vi "PLC Driver.vi"(0 "Data Cluster":T2={"Baud Rate"=9600, "Starting Address"=[], "Input Registers to write"=[], "No Of Inputs"=0, "Coils to write"=[], "VISA Port"=""} {"Starting Address" format="%.0x"}, 11 "Error in":errorcluster, 12 "Options":T1=enum."Initialize") -> (4 "register values":u16[](array[numeric]), 6 "Coils":bool[](array[boolean]), 8 "Object ID":string, 15 "Error out":errorcluster)   [LabVIEW 2022 SP3]
uses:
  Controls/Data.ctl
  Controls/Driver_States.ctl
  <vilib>/NI/Modbus Library/Master Function Definition/Read Device ID code.ctl
  <vilib>/NI/Modbus Library/API/Wrapper/Create Serial Master.vi
  <vilib>/NI/Modbus Library/API/Master/Modbus Master.lvclass
  <vilib>/NI/Modbus Library/Data Model/Device Data Model.lvclass
  <vilib>/NI/Modbus Library/API/Wrapper/API Main.lvlib
panel:
  # "Each PLC has its own operations to perform, Please refer to the PLC manual and choose its operations with its corresponding registers."
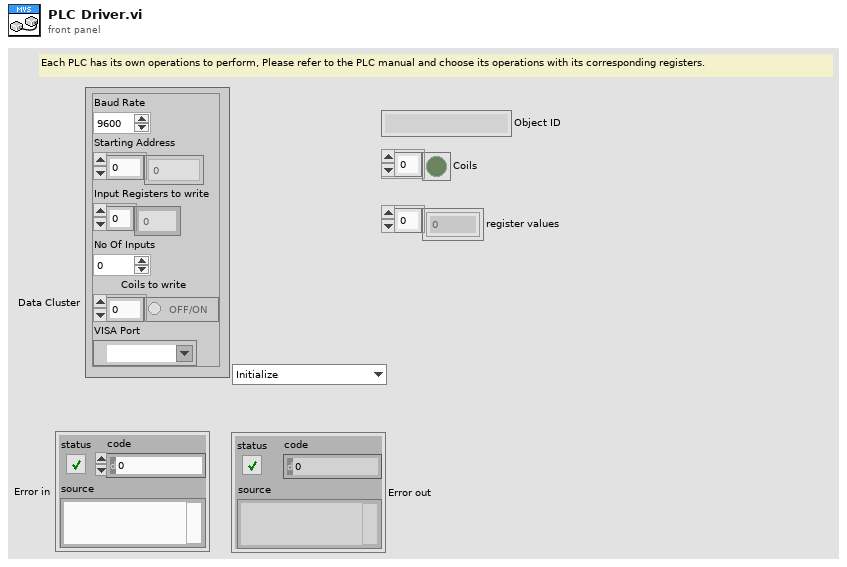
[diagram p1: front panel]
types:
  T1 = typedef "Driver_States.ctl" = enum16{"Poll", "Initialize", "Read Coil", "Read Multiple Coil", "Read Holding Register", "Read Multiple Holding Registers", "Read Multiple Register", "Write Single Coil", "Write Multiple Coils", "Write Multiple Register", "Read/Write", "Error", "Exit"}
  T2 = typedef "Data.ctl" = cluster{"Baud Rate":u16, "Starting Address":u16[], "Input Registers to write":u16[], "No Of Inputs":u16, "Coils to write":bool[], "VISA Port":refnum<visa-resource-name>}
  T3 = typedef "Device Data Model.lvclass/Read Device ID code.ctl" = enum8{"Read Basic", "Read Regular", "Read Extended", "Read Specific"}
  T4 = typedef "Device Data Model.lvclass/Identification Parameters.ctl" = cluster{"Object ID":u8, "Value":string}
  T5 = cluster{"objects[0]":T4, "objects[1]":T4, "objects[2]":T4, "objects[3]":T4, "objects[4]":T4, "objects[5]":T4, "objects[6]":T4, "objects[7]":T4, "objects[8]":T4}
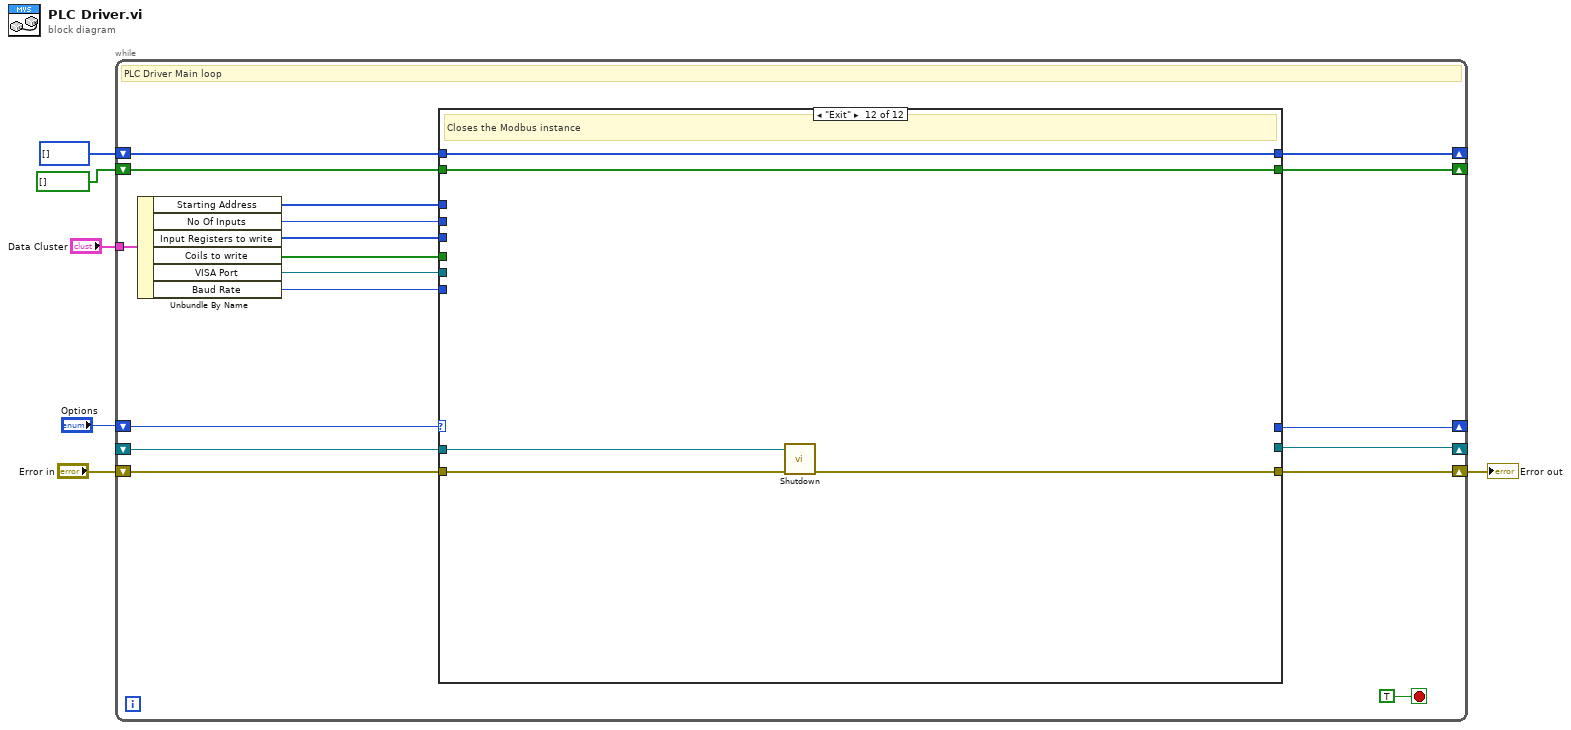
[diagram p0: block diagram]
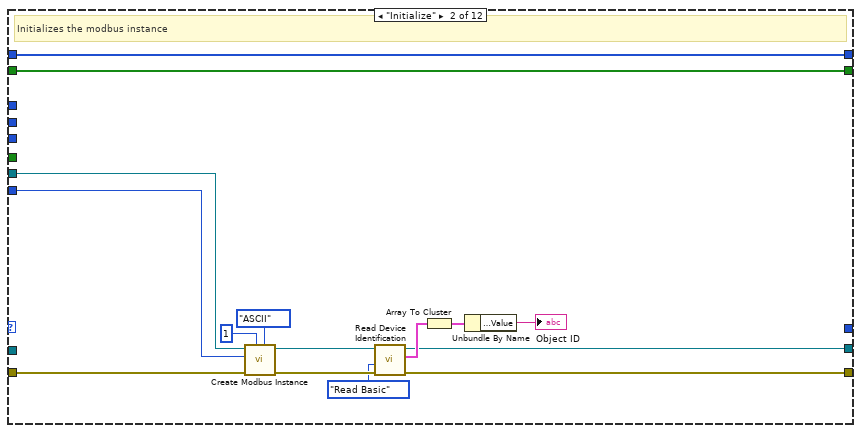
[diagram p3: hidden frame]
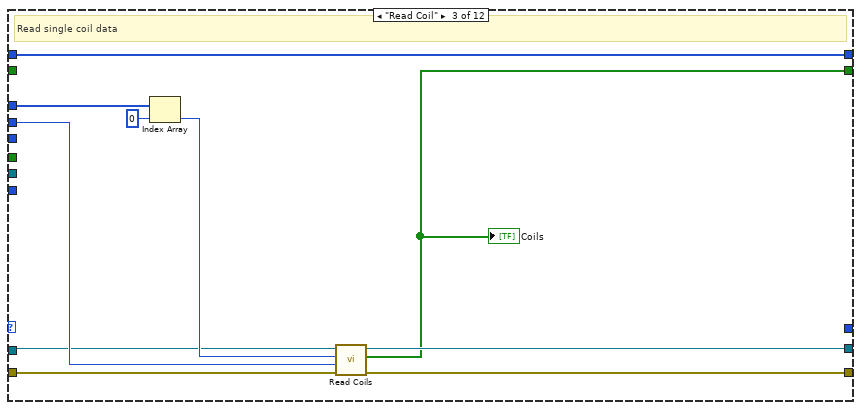
[diagram p4: hidden frame]
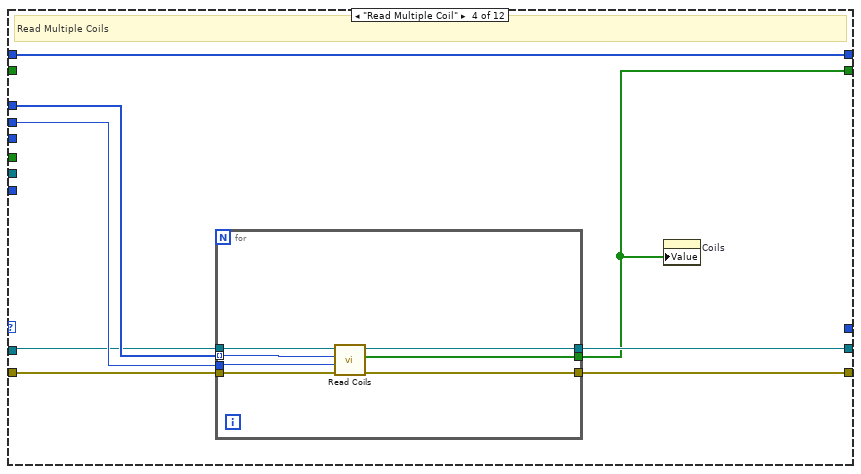
[diagram p5: hidden frame]
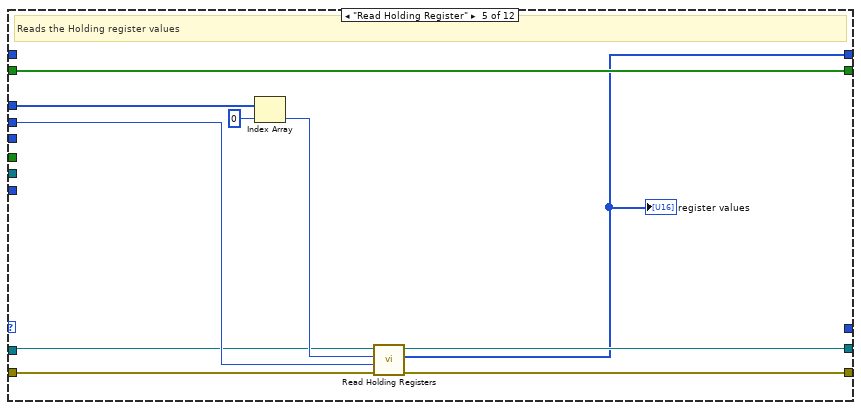
[diagram p6: hidden frame]
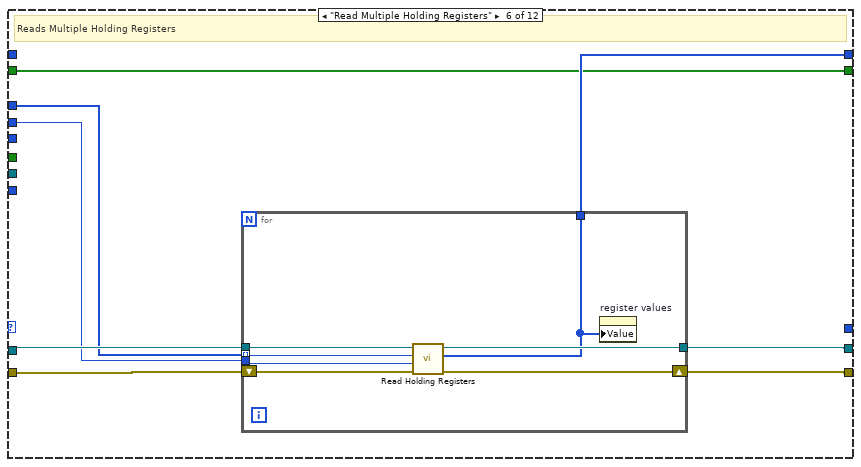
[diagram p7: hidden frame]
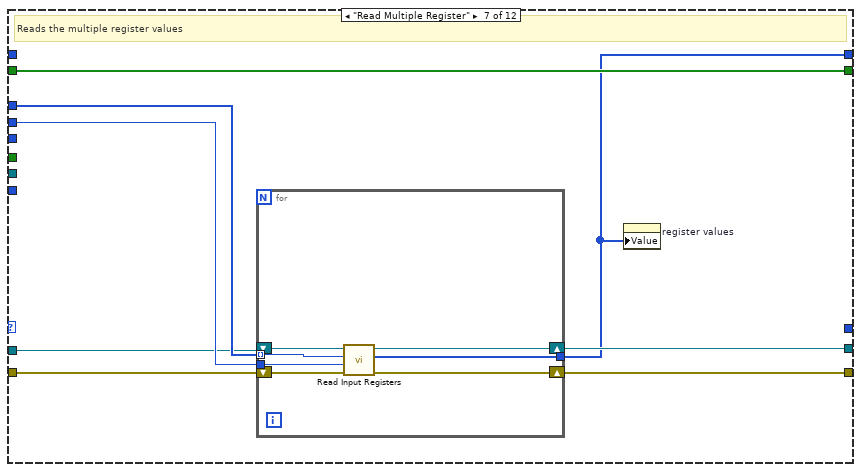
[diagram p8: hidden frame]
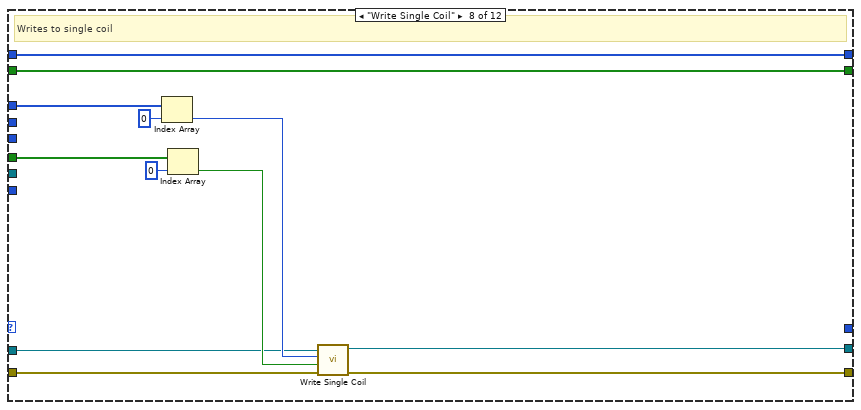
[diagram p9: hidden frame]
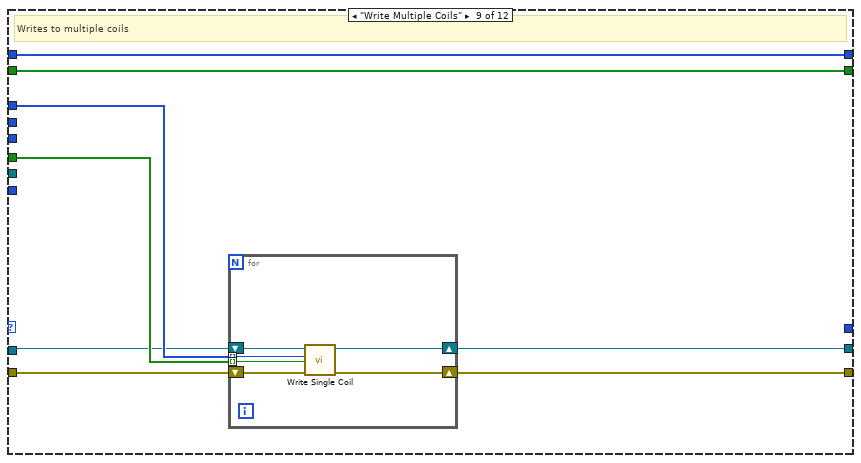
[diagram p10: hidden frame]
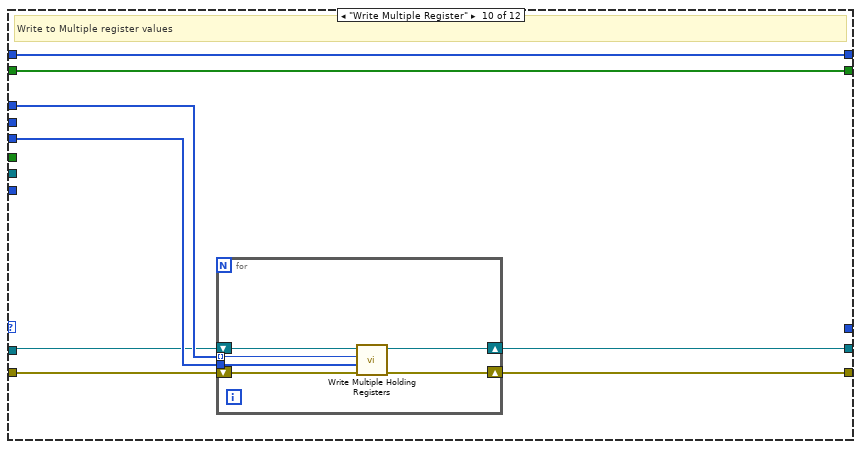
[diagram p11: hidden frame]
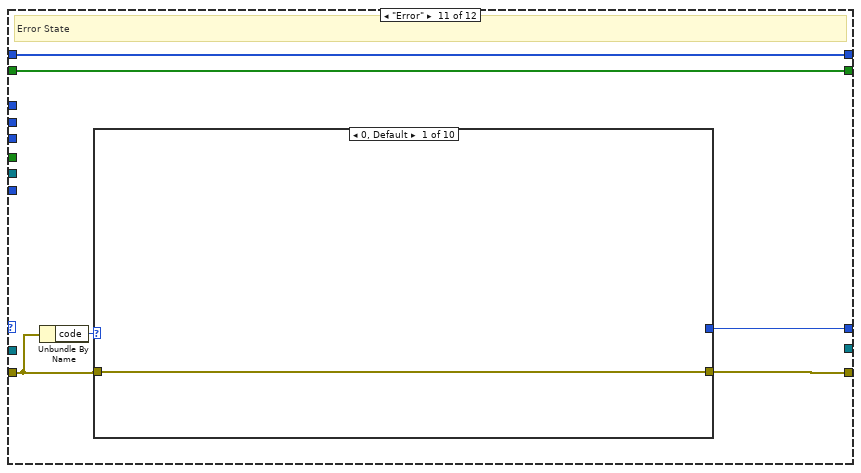
[diagram p12: hidden frame]
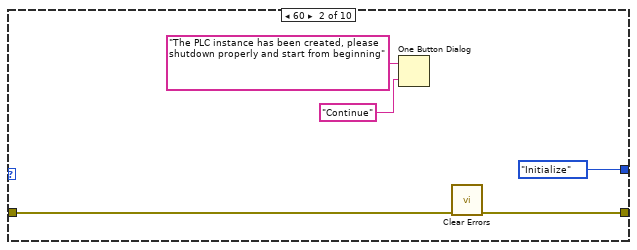
[diagram p13: hidden frame]
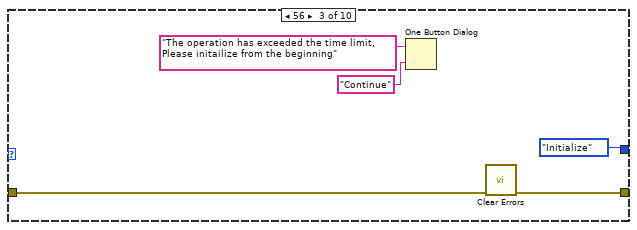
[diagram p14: hidden frame]
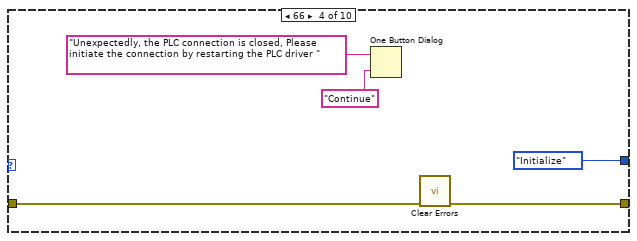
[diagram p15: hidden frame]
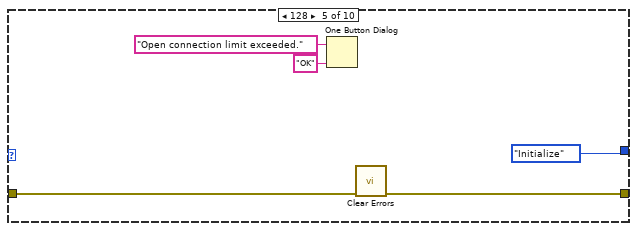
[diagram p16: hidden frame]
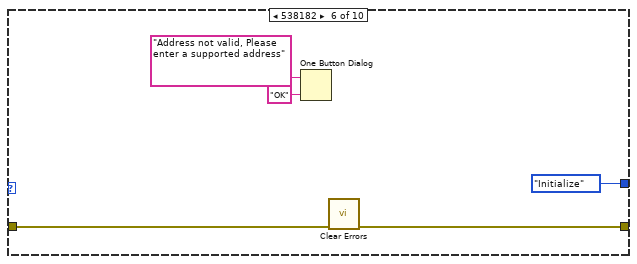
[diagram p17: hidden frame]
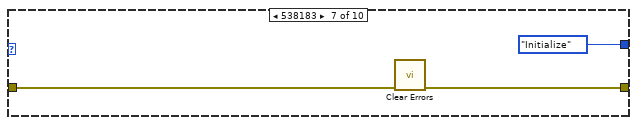
[diagram p18: hidden frame]
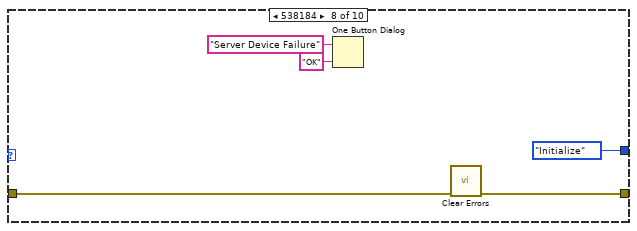
[diagram p19: hidden frame]
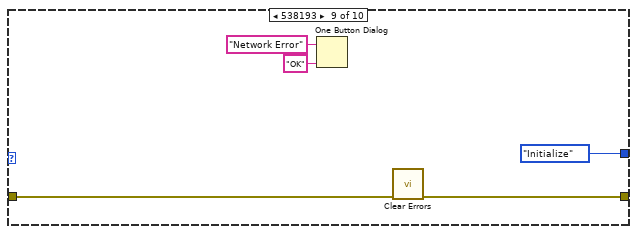
[diagram p20: hidden frame]
diagram:
  n1 = while {
    shift-right: [w12] -> w6
    shift-left: "Error in" -> [w15]
    shift-right: [w24] -> _
    shift-left: u16[] [] ("register values") -> [w22]
    shift-right: [w23] -> _
    shift-left: bool[] [] ("coils") -> [w21]
    tunnel: "Data Cluster" -> [w20]
    shift-right: [w9] -> _
    shift-left: "Options" -> [w10]
    shift-right: [w11] -> _
    shift-left: _ -> [w13]
    stop <- TRUE stop-if-true
    # "PLC Driver Main loop"
    n2 = Unbundle By Name(w20) -> ("Starting Address"=w19:u16[], "No Of Inputs"=w18:u16, "Input Registers to write"=w17:u16[], "Coils to write"=w16:bool[], "VISA Port"=w7:refnum<visa-resource-name>, "Baud Rate"=w14:u16)
    n3 = case shown="\"Exit\"" w10 {
      tunnel: [w26 w35 w52 w61 w74 w85 w101 w120 w128 w142 w153 w200] -> w12
      tunnel: [w25 w34 w53 w60 w75 w84 w100 w119 w127 w141 _ _] -> w11
      tunnel: [w28 w32 w51 w59 w73 w80 w98 w117 w126 w140 w152 w203] -> w24
      tunnel: [w27 w33 w44 w56 w78 w79 w99 w118 w125 w139 w151 w202] -> w23
      tunnel: w22 -> [w28 w32 w51 w59 _ _ _ w117 w126 w140 w152 w203]
      tunnel: w21 -> [w27 w33 _ _ w78 w79 w99 w118 w125 w139 w151 w202]
      tunnel: [_ _ _ _ _ _ _ _ _ _ w149 _] -> w9
      tunnel: w19 -> [_ _ w49 w58 w76 w82 w96 w113 w123 w137 _ _]
      tunnel: w18 -> [_ _ w48 w57 w71 w81 w97 _ _ _ _ _]
      tunnel: w16 -> [_ _ _ _ _ _ _ w114 w124 _ _ _]
      tunnel: w17 -> [_ _ _ _ _ _ _ _ _ w138 _ _]
      tunnel: w15 -> [w26 w37 w45 w55 w70 w86 w94 w109 w122 w136 w150 w201]
      tunnel: w14 -> [_ w36 _ _ _ _ _ _ _ _ _ _]
      tunnel: w13 -> [w25 _ w46 w54 w69 w83 w95 w110 w121 w135 _ w199]
      tunnel: w7 -> [_ w29 _ _ _ _ _ _ _ _ _ _]
      frame "Poll", Default {
        # "Waits for the operation to be performed"
      }
      frame "Initialize" {
        # "Initializes the modbus instance"
        n4 = call-poly <vilib>:"Create Modbus Instance.vi"("serial type"=enum16{"RTU", "ASCII"}."ASCII", "unit ID"=u8 1, "error in"=w37, "baud rate"=w36, "VISA resource name"=w29) -> ("error out"=w42:errorcluster, "serial master instance"=w43:refnum<class "Modbus Master.lvclass">)  [unwired: 5 in]
        n5 = call-dynamic "Read Device Identification.vi"("error in"=w42, "read device ID code"=Read_Device_ID_code."Read Basic", "Modbus master in"=w43) -> ("error out"=w35:errorcluster, "objects"=w41:T4[], "Modbus master out"=w34:refnum<class "Modbus Master.lvclass">)  [unwired: 6 in]
        n6 = Array To Cluster(array=w41) -> (cluster=w40:T5)
        n7 = Unbundle By Name(w40) -> ("objects[0].Value"=→"Object ID":string)
      }
      frame "Read Coil" {
        # "Read single coil data"
        n8 = Index Array(array=w49, index=0) -> (element=w47:u16)
        n9 = call-dynamic "Read Coils.vi"("error in"=w45, "number of inputs"=w48, "starting address"=w47, "Modbus master in"=w46) -> ("error out"=w52:errorcluster, "coils"=w44:bool[], "Modbus master out"=w53:refnum<class "Modbus Master.lvclass">)  [unwired: 5 in]
        "Coils" <- w44
      }
      frame "Read Multiple Coil" {
        # "Read Multiple Coils"
        n10 = for {
          tunnel: [w68] -> w61
          tunnel: w55 -> [w67]
          tunnel: w54 -> [w66]
          tunnel: [w65] -> w60
          tunnel: [w64] -> w56
          tunnel: w58 -> [w63] mode=indexing
          tunnel: w57 -> [w62]
          n11 = call-dynamic "Read Coils.vi"("error in"=w67, "number of inputs"=w62, "starting address"=w63, "Modbus master in"=w66) -> ("error out"=w68:errorcluster, "coils"=w64:bool[], "Modbus master out"=w65:refnum<class "Modbus Master.lvclass">)  [unwired: 5 in]
        }
        n12 = property on="Coils" class="Arr (strict)"("Value"=w56) -> ()  [unwired: 2 in, 2 out]
      }
      frame "Read Holding Register" {
        # "Reads the Holding register values"
        n13 = Index Array(array=w76, index=0) -> (element=w72:u16)
        n14 = call-dynamic "Read Holding Registers.vi"("error in"=w70, "number of inputs"=w71, "starting address"=w72, "Modbus master in"=w69) -> ("error out"=w74:errorcluster, "register values"=w73:u16[], "Modbus master out"=w75:refnum<class "Modbus Master.lvclass">)  [unwired: 5 in]
        "register values" <- w73
      }
      frame "Read Multiple Holding Registers" {
        # "Reads Multiple Holding Registers"
        n15 = for {
          tunnel: [w91] -> w84
          tunnel: w83 -> [w90]
          shift-right: [w92] -> w85
          shift-left: w86 -> [w93]
          tunnel: w82 -> [w89] mode=indexing
          tunnel: w81 -> [w88]
          tunnel: [w87] -> w80
          n16 = call-dynamic "Read Holding Registers.vi"("error in"=w93, "number of inputs"=w88, "starting address"=w89, "Modbus master in"=w90) -> ("error out"=w92:errorcluster, "register values"=w87:u16[], "Modbus master out"=w91:refnum<class "Modbus Master.lvclass">)  [unwired: 5 in]
          n17 = property on="register values" class="Arr (strict)"("Value"=w87) -> ()  [unwired: 2 in, 2 out]
        }
      }
      frame "Read Multiple Register" {
        # "Reads the multiple register values"
        n18 = for {
          tunnel: w97 -> [w102]
          tunnel: [w104] -> w98
          shift-right: [w106] -> w100
          shift-left: w95 -> [w107]
          shift-right: [w108] -> w101
          shift-left: w94 -> [w105]
          tunnel: w96 -> [w103] mode=indexing
          n19 = call-dynamic "Read Input Registers.vi"("error in"=w105, "number of inputs"=w102, "starting address"=w103, "Modbus master in"=w107) -> ("error out"=w108:errorcluster, "register values"=w104:u16[], "Modbus master out"=w106:refnum<class "Modbus Master.lvclass">)  [unwired: 5 in]
        }
        n20 = property on="register values" class="Arr (strict)"("Value"=w98) -> ()  [unwired: 2 in, 2 out]
      }
      frame "Write Single Coil" {
        # "Writes to single coil"
        n21 = Index Array(array=w113, index=0) -> (element=w111:u16)
        n22 = Index Array(array=w114, index=0) -> (element=w112:bool)
        n23 = call-dynamic "Write Single Coil.vi"("error in"=w109, "coil to write"=w112, "address"=w111, "Modbus master in"=w110) -> ("error out"=w120:errorcluster, "Modbus master out"=w119:refnum<class "Modbus Master.lvclass">)  [unwired: 6 in]
      }
      frame "Write Multiple Coils" {
        # "Writes to multiple coils"
        n24 = for {
          tunnel: w123 -> [w130] mode=indexing
          shift-right: [w134] -> w128
          shift-left: w122 -> [w133]
          shift-right: [w131] -> w127
          shift-left: w121 -> [w132]
          tunnel: w124 -> [w129] mode=indexing
          n25 = call-dynamic "Write Single Coil.vi"("error in"=w133, "coil to write"=w129, "address"=w130, "Modbus master in"=w132) -> ("error out"=w134:errorcluster, "Modbus master out"=w131:refnum<class "Modbus Master.lvclass">)  [unwired: 6 in]
        }
      }
      frame "Write Multiple Register" {
        # "Write to Multiple register values"
        n26 = for {
          tunnel: w137 -> [w147] mode=indexing
          tunnel: w138 -> [w143]
          shift-right: [w145] -> w141
          shift-left: w135 -> [w146]
          shift-right: [w148] -> w142
          shift-left: w136 -> [w144]
          n27 = call-dynamic "Write Multiple Holding Registers.vi"("error in"=w144, "registers to write"=w143, "starting address"=w147, "Modbus master in"=w146) -> ("error out"=w148:errorcluster, "Modbus master out"=w145:refnum<class "Modbus Master.lvclass">)  [unwired: 6 in]
        }
      }
      frame "Error" {
        # "Error State"
        n28 = Unbundle By Name(w150) -> ("code"=w154:i32)
        n29 = case shown="0, Default" w154 {
          tunnel: w150 -> [w155 w157 w165 w170 w173 w177 w183 w188 w193 w198]
          tunnel: [w155 w160 w164 w167 w172 w178 w182 w187 w192 w197] -> w153
          tunnel: [_ Driver_States."Initialize" ("Options") Driver_States."Initialize" ("Options") Driver_States."Initialize" ("Options") Driver_States."Initialize" ("Options") Driver_States."Initialize" ("Options") Driver_States."Initialize" ("Options") Driver_States."Initialize" ("Options") Driver_States."Initialize" ("Options") Driver_States."Initialize" ("Options")] -> w149
          frame 0, Default {
          }
          frame 60 {
            n30 = One Button Dialog(message="The PLC instance has been created, please shutdown properly and start from beginning", button name ("OK")="Continue") -> ()  [unwired: 1 out]
            n31 = call <vilib>:"Clear Errors.vi"("error in (no error)"=w157) -> ("error out"=w160:errorcluster)  [unwired: 5 in, 1 out]
          }
          frame 56 {
            n32 = One Button Dialog(message="The operation has exceeded the time limit, Please initailize from the beginning", button name ("OK")="Continue") -> ()  [unwired: 1 out]
            n33 = call <vilib>:"Clear Errors.vi"("error in (no error)"=w165) -> ("error out"=w164:errorcluster)  [unwired: 5 in, 1 out]
          }
          frame 66 {
            n34 = One Button Dialog(message="Unexpectedly, the PLC connection is closed, Please initiate the connection by restarting the PLC driver ", button name ("OK")="Continue") -> ()  [unwired: 1 out]
            n35 = call <vilib>:"Clear Errors.vi"("error in (no error)"=w170) -> ("error out"=w167:errorcluster)  [unwired: 5 in, 1 out]
          }
          frame 128 {
            n36 = One Button Dialog(message="Open connection limit exceeded.", button name ("OK")="OK") -> ()  [unwired: 1 out]
            n37 = call <vilib>:"Clear Errors.vi"("error in (no error)"=w173) -> ("error out"=w172:errorcluster)  [unwired: 5 in, 1 out]
          }
          frame 538182 {
            n38 = One Button Dialog(message="Address not valid, Please enter a supported address", button name ("OK")="OK") -> ()  [unwired: 1 out]
            n39 = call <vilib>:"Clear Errors.vi"("error in (no error)"=w177) -> ("error out"=w178:errorcluster)  [unwired: 5 in, 1 out]
          }
          frame 538183 {
            n40 = call <vilib>:"Clear Errors.vi"("error in (no error)"=w183) -> ("error out"=w182:errorcluster)  [unwired: 5 in, 1 out]
          }
          frame 538184 {
            n41 = One Button Dialog(message="Server Device Failure", button name ("OK")="OK") -> ()  [unwired: 1 out]
            n42 = call <vilib>:"Clear Errors.vi"("error in (no error)"=w188) -> ("error out"=w187:errorcluster)  [unwired: 5 in, 1 out]
          }
          frame 538193 {
            n43 = One Button Dialog(message="Network Error", button name ("OK")="OK") -> ()  [unwired: 1 out]
            n44 = call <vilib>:"Clear Errors.vi"("error in (no error)"=w193) -> ("error out"=w192:errorcluster)  [unwired: 5 in, 1 out]
          }
          frame 538179 {
            n45 = One Button Dialog(message="The device has not been initialised, Please initialise the Modbus instance and then proceed", button name ("OK")="OK") -> ()  [unwired: 1 out]
            n46 = call <vilib>:"Clear Errors.vi"("error in (no error)"=w198) -> ("error out"=w197:errorcluster)  [unwired: 5 in, 1 out]
          }
        }
      }
      frame "Exit" {
        # "Closes the Modbus instance"
        n47 = call-dynamic "Shutdown.vi"("error in"=w201, "Modbus master in"=w199) -> ("error out"=w200:errorcluster)  [unwired: 9 in]
      }
    }
  }
  "Error out" <- w6
